vi "Install.vi"() -> ()   [LabVIEW 2014]
panel:
  out "error out":errorcluster
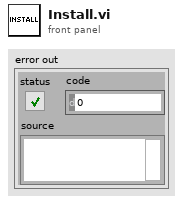
[diagram p1: front panel]
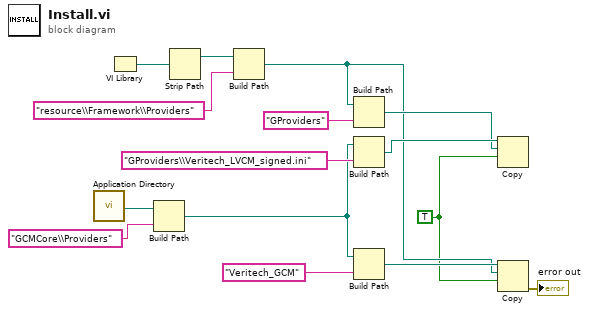
[diagram p0: block diagram]
diagram:
  w2 = TRUE ("overwrite (F)")
  n1 = call <vilib>:"Application Directory.vi"() -> ("Application Directory"=w15:path)
  n2 = VI Library() -> (path=w11:path)
  n3 = Build Path(base path=w15, name or relative path="GCMCore\\Providers") -> (appended path=w6:path)
  n4 = Strip Path(path=w11) -> (stripped path=w10:path)  [unwired: 1 out]
  n5 = Build Path(base path=w10, name or relative path="resource\\Framework\\Providers") -> (appended path=w3:path)
  n6 = Build Path(base path=w3, name or relative path="GProviders") -> (appended path=w7:path)
  n7 = Build Path(base path=w6, name or relative path="GProviders\\Veritech_LVCM_signed.ini") -> (appended path=w12:path)
  n8 = Build Path(base path=w6, name or relative path="Veritech_GCM") -> (appended path=w4:path)
  n9 = Copy(9:w2, 10:w7, 11:w12) -> ()  [unwired: 2 in, 3 out]
  n10 = Copy(9:w2, 10:w3, 11:w4) -> (0:→"error out":errorcluster)  [unwired: 2 in, 2 out]
